vi "Stop.vi"(8 "error in (no error)":errorcluster, 11 "Cache Manager DVR in":refnum<class "Cache Manager.lvclass">) -> (0 "error out":errorcluster, 3 "Cache Manager DVR out":refnum<class "Cache Manager.lvclass">)   [LabVIEW 2020, in "Cache Manager.lvclass"]
uses:
  Cache Manager.lvclass
  Cache Manager.lvclass/Cache Manager.ctl
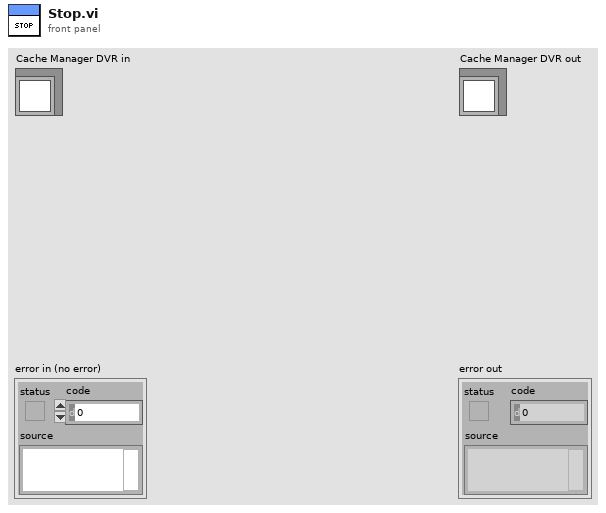
[diagram p1: front panel]
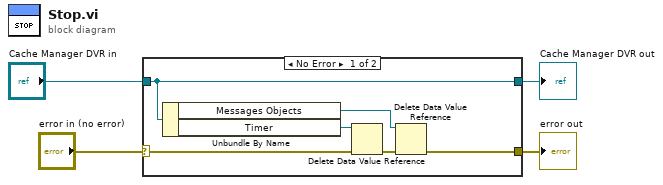
[diagram p0: block diagram]
diagram:
  n1 = case shown="No Error" "error in (no error)" {
    selector: "error in (no error)" -> [w8 w12]
    tunnel: [w5 w12] -> w3
    tunnel: [w10 w11] -> w1
    tunnel: "Cache Manager DVR in" -> [w10 w11]
    frame No Error {
      n2 = Unbundle By Name(w10) -> ("Messages Objects"=w6:refnum<data-value>, "Timer"=w7:refnum<data-value>)
      n3 = Delete Data Value Reference(data value reference=w7, error in=w8) -> (error out=w9:errorcluster)  [unwired: 1 out]
      n4 = Delete Data Value Reference(data value reference=w6, error in=w9) -> (error out=w5:errorcluster)  [unwired: 1 out]
    }
    frame Error {
    }
  }
  "error out" <- w3
  "Cache Manager DVR out" <- w1
